vi "LVObject to JSON.vi"(7 "Flatten To JSON Object in":refnum<class "Flatten To JSON Object.lvclass">, 8 "error in (no error)":errorcluster, 10 "Object":refnum<class>) -> (0 "error out":errorcluster, 2 "<JSON>Object":string)   [LabVIEW 2017, in "Flatten To JSON Object.lvclass"]
uses:
  Flatten To JSON Object.lvclass
  C:/Program Files (x86)/National Instruments/LabVIEW 2017/vi.lib/JDP Science/JSONtext/LVClass Serializer/JSONtext LVClass Serializer.lvclass
  <vilib>/JDP Science/JSONtext/Get all Object Items.vi
  <vilib>/JDP Science/JSONtext/Set Multiple Object Items.vi
  <vilib>/PNR/LabVIEW Composition/Composition/Composition.lvlib
  <vilib>/JDP Science/JSONtext/JSONtext.lvlib
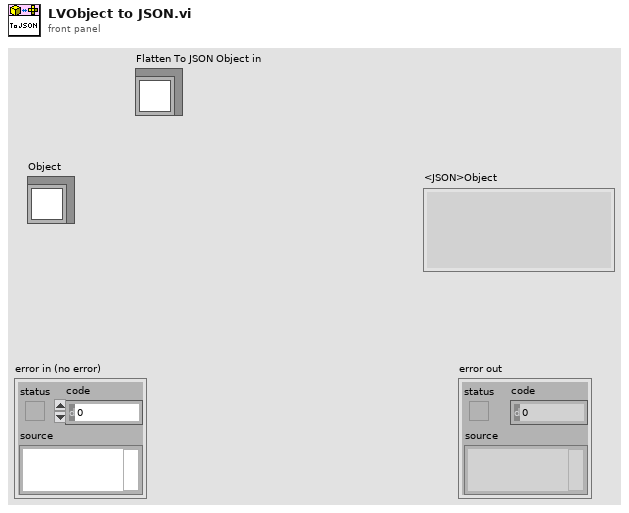
[diagram p1: front panel]
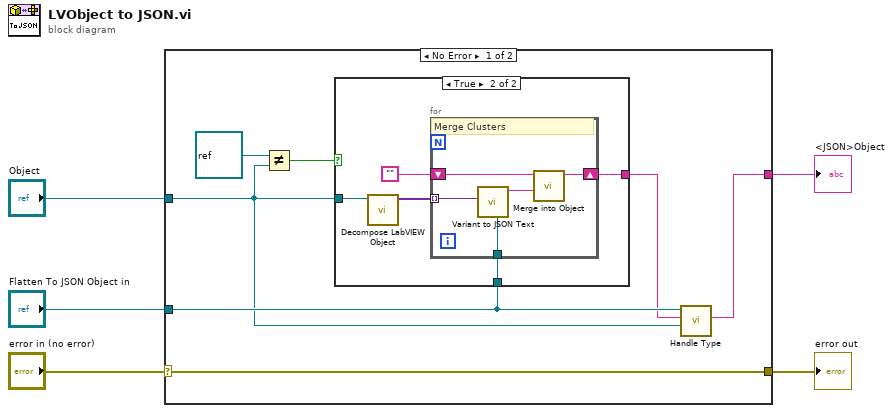
[diagram p0: block diagram]
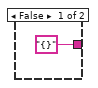
[diagram p2: hidden frame]
diagram:
  n1 = case shown="No Error" "error in (no error)" {
    selector: "error in (no error)" -> [w10 w24]
    tunnel: "Object" -> [w8 _]
    tunnel: [w6 _] -> w4
    tunnel: "Flatten To JSON Object in" -> [w9 _]
    tunnel: [w10 w24] -> w1
    frame No Error {
      n2 = Not Equal?(x=refnum<class> refnum, y=w8) -> (x != y?=w11:bool)
      n3 = case shown="True" w11 {
        tunnel: ["{}" ("<JSON>") w15] -> w7
        tunnel: w8 -> [_ w18]
        tunnel: w9 -> [_ w14]
        frame False {
        }
        frame True {
          n4 = call <vilib>:"Decompose LabVIEW Object.vi"("LabVIEW Object"=w18) -> ("Private Data Clusters"=w17:variant[])  [unwired: 7 in, 3 out]
          n5 = for {
            tunnel: w17 -> [w23] mode=indexing
            shift-right: [w20] -> w15
            shift-left: "" -> [w21]
            tunnel: w14 -> [w19]
            # "Merge Clusters"
            n6 = call <vilib>:"Variant to JSON Text.vi"("LVClass Serializer"=w19, "Variant"=w23) -> ("<JSON>"=w22:string)  [unwired: 7 in, 2 out]
            n7 = call <vilib>:"Merge into Object.vi"("JSON Object to Merge"=w22, "JSON"=w21) -> ("<JSON>"=w20:string)  [unwired: 7 in, 1 out]
          }
        }
      }
      n8 = call "Handle Type.vi"("Type"=w8, "JSON"=w7, "Flatten To JSON Object in"=w9) -> ("JSON out"=w6:string)  [unwired: 6 in, 2 out]
    }
    frame Error {
    }
  }
  "error out" <- w1
  "<JSON>Object" <- w4
